vi "Open HP3488A Switcher(GPIB).vi"(0 "Device In":cluster{"GPIB":u8, "Address":u8}={"GPIB"=1, "Address"=6} {"Address" min=1 max=31; "GPIB" min=1 max=5}, 1 "reset":bool, 3 "Use Card# 5":bool, 4 "ID query":bool, 5 "error in (no error)":errorcluster, 6 "Position Number":u8=1 min=1 max=40 step=1) -> (7 "error out":errorcluster)   [LabVIEW 2023]
uses:
  Agilent 3488/Agilent 3488.lvlib
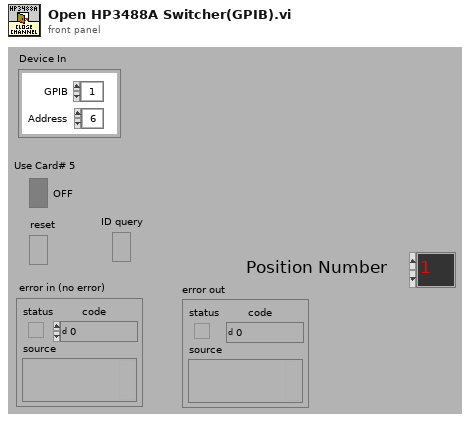
[diagram p1: front panel]
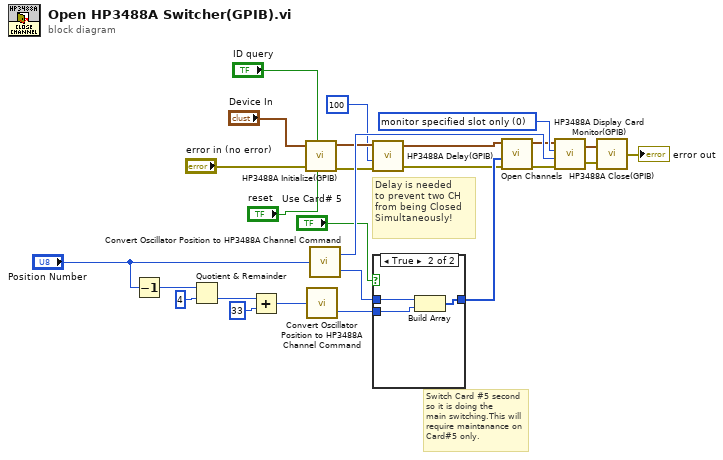
[diagram p0: block diagram]
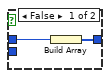
[diagram p2: hidden frame]
diagram:
  w6 = u16 0 items=["monitor specified slot only", "monitor tracking mode starting with specified slot", "card monitor off"] ("card monitor (2: off)")
  # "Switch Card #5 second\nso it is doing the\nmain switching.This will\nrequire maintanance on\nCard#5 only."
  # "Delay is needed \nto prevent two CH\nfrom being Closed \nSimultaneously!"
  n1 = Decrement(x="Position Number") -> (x-1=w20:u8)
  n2 = Quotient & Remainder(x=w20, y=u8 4) -> (floor(x/y)=w18:u8)  [unwired: 1 out]
  n3 = Add(x=w18, y=u8 33) -> (x+y=w16:u8)
  n4 = call "HP3488A Initialize(GPIB).vi"("Device In"="Device In", "ID query"="ID query", "error in (no error)"="error in (no error)", "reset"="reset") -> ("Device Out"=w9:cluster{"GPIB":u8, "Address":u8}, "error out"=w22:errorcluster)  [unwired: 3 in]
  n5 = call "Convert Oscillator Position to HP3488A Channel Command.vi"("Position Number"=w16) -> ("HP3488A Position Code"=w15:i16)  [unwired: 3 out]
  n6 = call "Convert Oscillator Position to HP3488A Channel Command.vi"("Position Number"="Position Number") -> ("HP3488A Position Code"=w14:i16, "Card#"=w25:i8)  [unwired: 2 out]
  n7 = call "HP3488A Delay(GPIB).vi"("error in (no error)"=w22, "set delay (0 ms)"=100, "Device In"=w9) -> ("error out"=w4:errorcluster, "Device Out"=w2:cluster{"GPIB#":i8, "Address":i8})  [unwired: 1 in, 1 out]
  n8 = case shown="True" "Use Card# 5" {
    tunnel: w15 -> [_ w29]
    tunnel: w14 -> [w27 w30]
    tunnel: [w28 w31] -> w5
    frame False {
      n9 = Build Array(w27) -> (w28:i16[])
    }
    frame True {
      n10 = Build Array(w30, w29) -> (w31:i16[])
    }
  }
  n11 = call "Open Channels.vi"("error in (no error)"=w4, "channel addresses"=w5, "Device In"=w2) -> ("error out"=w3:errorcluster, "Device Out"=w1:cluster{"GPIB":u8, "Address":u8})  [unwired: 7 in]
  n12 = call "HP3488A Display Card Monitor(GPIB).vi"("error in (no error)"=w3, "slot number (1)"=w25, "card monitor (2: off)"=w6, "Device In"=w1) -> ("error out"=w24:errorcluster, "Device Out"=w7:cluster{"GPIB":u8, "Address":u8})
  n13 = call "HP3488A Close(GPIB).vi"("error in (no error)"=w24, "Device In"=w7) -> ("error out"=→"error out":errorcluster)
